vi "Nest Msg Q Alias.vi"(8 "error in (no error)":errorcluster, 11 "Self Actor in":refnum<class "Self Actor.lvclass">) -> (0 "error out":errorcluster, 3 "Self Actor out":refnum<class "Self Actor.lvclass">)   [LabVIEW 2021, in "LVCAM.lvlib" / "Self Actor.lvclass"]
uses:
  Self Actor.lvclass
  LVCAM/LVCAM.lvclass
  Self Actor.lvclass/Self Actor.ctl
  Msg Q/Msg Q.lvclass
panel:
  out "Alias found?":bool
  in  "Alias":string
  in  "Self Actor":refnum<class "LVCAM.lvclass">
  out "Nest Actor Aliases":string[](array[string])
  out "error out 2":errorcluster
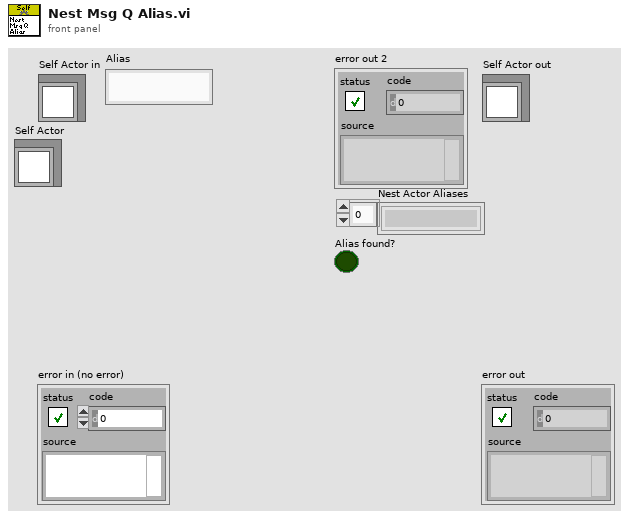
[diagram p1: front panel]
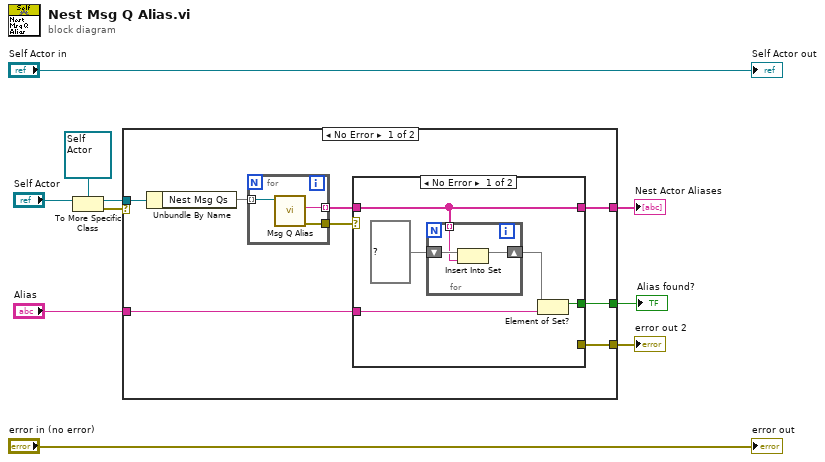
[diagram p0: block diagram]
diagram:
  n1 = To More Specific Class(target class=refnum<class "Self Actor.lvclass"> refnum ("LVCAM.lvlib:Self Actor.lvclass"), reference="Self Actor") -> (specific class reference=w5:refnum<class "Self Actor.lvclass">, error out=w3:errorcluster)  [unwired: 1 in]
  n2 = case shown="No Error" w3 {
    selector: w3 -> [_ w31]
    tunnel: [w15 w31] -> w8
    tunnel: [w14 _] -> w7
    tunnel: w5 -> [w17 _]
    tunnel: "Alias" -> [w12 _]
    tunnel: [w11 _] -> w1
    frame No Error {
      n3 = Unbundle By Name(w17) -> ("Nest Msg Qs"=w18:set{refnum<class "Msg Q.lvclass">})
      n4 = for {
        tunnel: w18 -> [w30] mode=indexing
        tunnel: [w29] -> w13 mode=indexing
        tunnel: [w28] -> w16
        n5 = call "Msg Q Alias.vi"("Msg Q in"=w30) -> ("error out"=w28:errorcluster, "Msg Q Alias"=w29:string)  [unwired: 9 in]
      }
      n6 = case shown="No Error" w16 {
        selector: w16 -> [_ w27]
        tunnel: [_ w27] -> w15
        tunnel: [w20 _] -> w14
        tunnel: w13 -> [w20 _]
        tunnel: w12 -> [w21 _]
        tunnel: [w19 _] -> w11
        frame No Error {
          n7 = for {
            tunnel: w20 -> [w24] mode=indexing
            shift-right: [w26] -> w22
            shift-left: set{string} {} ("empty set") -> [w25]
            n8 = Insert Into Set(10:w24, 11:w25) -> (3:w26:set{string})  [unwired: 1 out]
          }
          n9 = Element of Set?(10:w21, 11:w22) -> (3:w19:bool)
        }
        frame Error {
          # "#LVCAMError"
        }
      }
    }
    frame Error {
    }
  }
  "error out 2" <- w8
  "Nest Actor Aliases" <- w7
  "Alias found?" <- w1
  "error out" <- "error in (no error)"
  "Self Actor out" <- "Self Actor in"
